vi "Init Command.vi"(5 "Sequencer":refnum<class "MessageQ.lvclass">, 6 "Variables":refnum<class "Variables.lvclass">, 7 "VolatusAPI":refnum<class "VolatusAPI.lvclass">, 8 "error in (no error)":refnum<class "MultiErrors.lvclass">, 10 "Command Config":refnum<class "Command Config.lvclass">, 11 "Stop Seq Command in":refnum<class "Stop Seq Command.lvclass">) -> (0 "error out":refnum<class "MultiErrors.lvclass">, 3 "Stop Seq Command out":T1)   [LabVIEW 2020, in "VolatusSeq.lvlib" / "Stop Seq Command.lvclass"]
uses:
  Stop Seq Command.lvclass
  VolatusErrorUtilities/MultiErrors/MultiErrors.lvclass
  Command.ctl
  Volatus/MessageQ/MessageQ.lvclass
  VolatusSeqConfig/Command Type.ctl
  messages/CmdDigital/Data.ctl
  messages/CmdAnalog/Data.ctl
  Send Type.ctl
  Volatus/VolatusAPI/VolatusAPI.lvclass
  VolatusSeqConfig/Command Config/Command Config.lvclass
  VolatusSeqConfig/Stop Seq Command Config/Stop Seq Command Config.lvclass
  Stop Seq Command.lvclass/Stop Seq Command.ctl
  VolatusSeqConfig/VolatusSeqConfig.lvlib
  VolatusSeq.lvlib
  messages/CmdAnalog/CmdAnalog.lvlib
  messages/CmdDigital/CmdDigital.lvlib
  Variables/Variables.lvclass
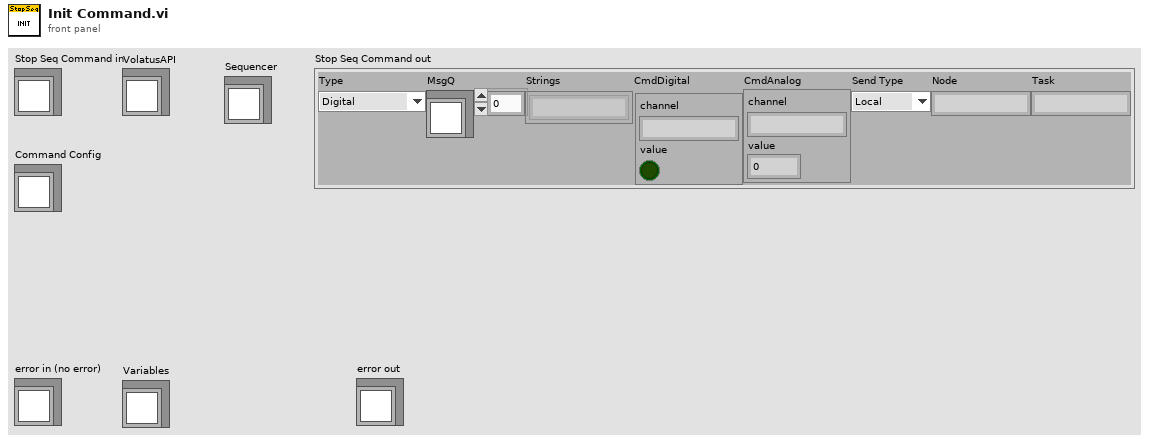
[diagram p1: front panel]
types:
  T1 = typedef "VolatusSeq.lvlib/Command.ctl" = cluster{"Type":T2, "MsgQ":refnum<class "MessageQ.lvclass">, "Strings":string[], "CmdDigital":T3, "CmdAnalog":T4, "Send Type":T5, "Node":string, "Task":string}
  T2 = typedef "VolatusSeqConfig.lvlib/Command Type.ctl" = enum16{"Digital", "Numeric", "Transition", "Stop", "StartLog", "StopLog", "Start", "Event", "Error", "HTTP"}
  T3 = typedef "CmdDigital.lvlib/Data.ctl" = cluster{"channel":string, "value":bool}
  T4 = typedef "CmdAnalog.lvlib/Data.ctl" = cluster{"channel":string, "value":dbl}
  T5 = typedef "VolatusSeq.lvlib/Send Type.ctl" = enum16{"Local", "Remote"}
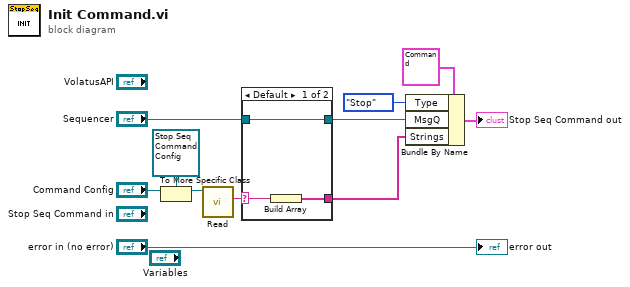
[diagram p0: block diagram]
diagram:
  n1 = To More Specific Class(target class=refnum<class "Stop Seq Command Config.lvclass"> refnum ("VolatusSeqConfig.lvlib:Stop Seq Command Config.lvclass"), reference="Command Config") -> (specific class reference=w5:refnum<class "Stop Seq Command Config.lvclass">)  [unwired: 1 in, 1 out]
  n2 = call "Read.vi"("Stop Seq Command Config in"=w5) -> ("Sequence"=w4:string)  [unwired: 8 in, 2 out]
  n3 = case shown="Default" w4 {
    selector: w4 -> [w14 _]
    tunnel: [w13 _] -> w3
    tunnel: "Sequencer" -> [w12 _]
    tunnel: [w12 _] -> w1
    frame Default {
      n4 = Build Array(w14) -> (w13:string[])
    }
    frame "" {
    }
  }
  n5 = Bundle By Name(cluster=T1 {"Type"=enum."Digital", "MsgQ"=refnum, "Strings"=[], "CmdDigital"={"channel"="", "value"=FALSE}, "CmdAnalog"={"channel"="", "value"=0.0}, "Send Type"=enum."Local", "Node"="", "Task"=""} ("Stop Seq Command out"), "Type"=Command_Type."Stop", "MsgQ"=w1, "Strings"=w3) -> (→"Stop Seq Command out":T1)
  "error out" <- "error in (no error)"
